vi "Instrument Get Free.vi"(4 "error in (no error)":errorcluster, 7 "Connection Refnum":T1) -> (0 "error out":errorcluster, 2 "Free Instruments":T2[](array[typedef]), 3 "Connection Refnum":T1)   [LabVIEW 2011]
uses:
  SI.LIB/ODBC/SQL Controls/Connection Refnum.ctl
  Instrument Record.ctl
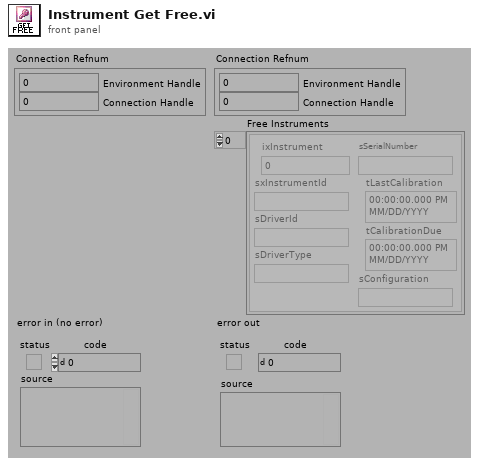
[diagram p1: front panel]
types:
  T1 = typedef "Connection Refnum.ctl" = cluster{"Environment Handle":i32, "Connection Handle":i32}
  T2 = typedef "Instrument Record.ctl" = cluster{"ixInstrument":i32, "sxInstrumentId":string, "sDriverId":string, "sDriverType":string, "sSerialNumber":string, "tLastCalibration":timestamp, "tCalibrationDue":timestamp, "sConfiguration":string}
  T3 = typedef "Association Record.ctl" = cluster{"ixAssociation":i32, "iStation":i32, "iInstrument":i32}
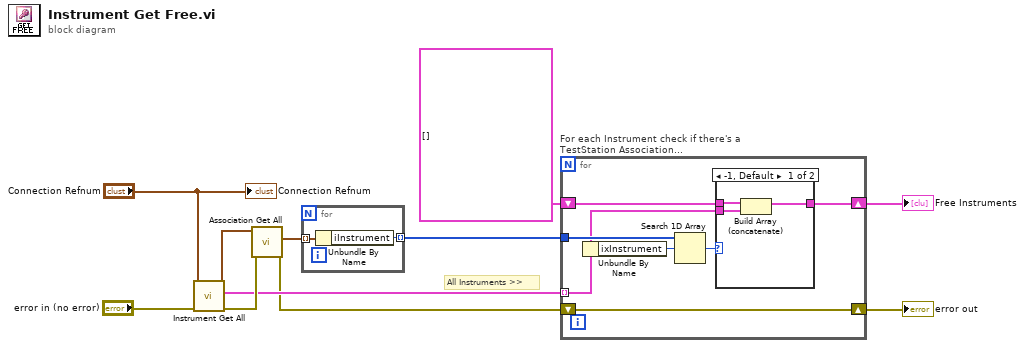
[diagram p0: block diagram]
diagram:
  # "All Instruments >>"
  n1 = call "Instrument Get All.vi"("error in (no error)"="error in (no error)", "Connection Refnum"="Connection Refnum") -> ("error out"=w10:errorcluster, "Instruments"=w8:T2[], "Connection Refnum"=w11:T1)  [unwired: 2 in, 5 out]
  n2 = call "Association Get All.vi"("error in (no error)"=w10, "Connection Refnum"=w11) -> ("error out"=w7:errorcluster, "Associations"=w5:T3[])  [unwired: 8 out]
  n3 = for {
    tunnel: w5 -> [w13] mode=indexing
    tunnel: [w12] -> w4 mode=indexing
    n4 = Unbundle By Name(w13) -> ("iInstrument"=w12:i32)
  }
  n5 = for "For each Instrument check if there's a TestStation Association..." {
    tunnel: w8 -> [w14] mode=indexing
    shift-right: [w18] -> w6
    shift-left: w7 -> [w18]
    tunnel: w4 -> [w20]
    shift-right: [w15] -> w2
    shift-left: T2[] [] ("Instruments") -> [w16]
    n6 = Unbundle By Name(w14) -> ("ixInstrument"=w19:i32)
    n7 = Search 1D Array(1D array=w20, element=w19) -> (index of element=w17:i32)  [unwired: 1 out]
    n8 = case shown="-1, Default" w17 {
      tunnel: w16 -> [w23 w24]
      tunnel: [w22 w24] -> w15
      tunnel: w14 -> [w21 _]
      frame -1, Default {
        n9 = Build Array (concatenate)(w23, w21) -> (w22:T2[])
      }
      frame 0.. {
      }
    }
  }
  "error out" <- w6
  "Free Instruments" <- w2
  "Connection Refnum" <- "Connection Refnum"
